vi "Set Scan Engine Mode.vi"(0 "target address (localhost)":string="localhost", 5 "mode (Active Mode)":i32(ring)=2 items=["Configuration Mode"=1, "Active Mode"=2], 11 "error in (no error)":errorcluster) -> (15 "error out":errorcluster)   [LabVIEW 2020]
doc: "Sets the operating mode of the NI Scan Engine on the target."
uses:
  <resource>/objmgr/ni.var.rc
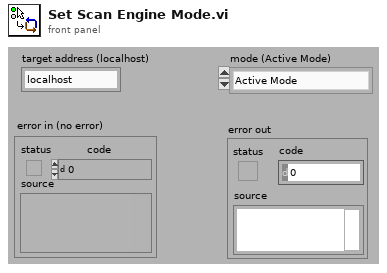
[diagram p1: front panel]
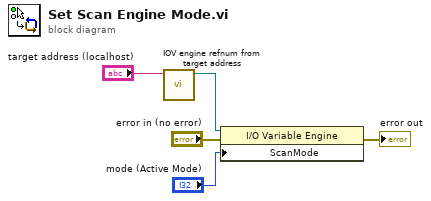
[diagram p0: block diagram]
diagram:
  n1 = call <vilib>:"IOV engine refnum from target address.vi"("target address"="target address (localhost)") -> ("reference out"=w4:refnum<k21>)  [unwired: 10 in]
  n2 = property class="I/O Variable Engine"(reference=w4, error in="error in (no error)", "ScanMode"="mode (Active Mode)") -> (error out=→"error out":errorcluster)  [unwired: 1 out]
